vi "Lab Panel V6.00.vi"() -> ()   [LabVIEW 2017] (continued)
                          }
                          frame #1 {
                            n1486 = Bundle(cluster=w2775, "STATUS"="T-RISE PASS") -> (w2777:T4)  [unwired: 2 in]
                            n1487 = local write "RESULT LAB04-1"(TRUE) -> ()
                            n1488 = local write "DISP LAB04-1"(w2777) -> ()
                          }
                        }
                      }
                      frame False {
                      }
                    }
                  }
                }
              }
              frame #7 {
                # "LAB04-2"
                n1489 = Equal?(x=w2780, y=2) -> (x = y?=w2783:bool)
                n1490 = local read "DISP LAB04-2"() -> (w2785:T4)
                n1491 = Unbundle(w2785) -> ("STATUS"=w2786:string)  [unwired: 2 out]
                n1492 = Equal?(x=w2786, y="RUN") -> (x = y?=w2782:bool)
                n1493 = And(x=w2782, y=w2783) -> (x .and. y?=w2781:bool)
                n1494 = case shown="True" w2781 {
                  tunnel: w2785 -> [_ w2789]
                  tunnel: w2779 -> [_ w2792]
                  frame False {
                  }
                  frame True {
                    n1495 = local read "SET LAB04-2"() -> (w2791:T5)
                    n1496 = local read "TDMS LAB04-2"() -> (w2788:refnum<k34>)
                    n1497 = Unbundle(w2789) -> ("CYCLE"=w2793:dbl)  [unwired: 2 out]
                    n1498 = Unbundle(w2791) -> ("T-RISE mins"=w2790:dbl)  [unwired: 4 out]
                    n1499 = Greater Or Equal?(x=w2793, y=w2792) -> (x >= y?=w2794:bool)
                    n1500 = case shown="True" w2794 {
                      tunnel: w2790 -> [w2797 _]
                      tunnel: w2789 -> [w2796 _]
                      tunnel: w2788 -> [w2795 _]
                      frame True {
                        n1501 = stacked-sequence {
                          tunnel: w2797 -> [w2800 _]
                          tunnel: w2796 -> [_ w2805]
                          tunnel: w2795 -> [w2798 _]
                          frame #0 {
                            n1502 = Build Array("T-RISE") -> (w2802:string[])
                            n1503 = Build Array(w2800) -> (w2801:dbl[])
                            n1504 = TDMS Write(0:w2798, 5:"TEST PASS", 7:w2802, 9:w2801) -> (15:w2804:errorcluster)  [unwired: 2 in, 3 out]
                            n1505 = local write "data file error"(w2804) -> ()
                          }
                          frame #1 {
                            n1506 = Bundle(cluster=w2805, "STATUS"="T-RISE PASS") -> (w2807:T4)  [unwired: 2 in]
                            n1507 = local write "RESULT LAB04-2"(TRUE) -> ()
                            n1508 = local write "DISP LAB04-2"(w2807) -> ()
                          }
                        }
                      }
                      frame False {
                      }
                    }
                  }
                }
              }
              frame #8 {
                # "LAB05-1"
                n1509 = Equal?(x=w2810, y=2) -> (x = y?=w2813:bool)
                n1510 = local read "DISP LAB05-1"() -> (w2815:T4)
                n1511 = Unbundle(w2815) -> ("STATUS"=w2816:string)  [unwired: 2 out]
                n1512 = Equal?(x=w2816, y="RUN") -> (x = y?=w2812:bool)
                n1513 = And(x=w2812, y=w2813) -> (x .and. y?=w2811:bool)
                n1514 = case shown="True" w2811 {
                  tunnel: w2815 -> [_ w2819]
                  tunnel: w2809 -> [_ w2822]
                  frame False {
                  }
                  frame True {
                    n1515 = local read "SET LAB05-1"() -> (w2821:T5)
                    n1516 = local read "TDMS LAB05-1"() -> (w2818:refnum<k34>)
                    n1517 = Unbundle(w2819) -> ("CYCLE"=w2823:dbl)  [unwired: 2 out]
                    n1518 = Unbundle(w2821) -> ("T-RISE mins"=w2820:dbl)  [unwired: 4 out]
                    n1519 = Greater Or Equal?(x=w2823, y=w2822) -> (x >= y?=w2824:bool)
                    n1520 = case shown="True" w2824 {
                      tunnel: w2820 -> [w2827 _]
                      tunnel: w2819 -> [w2826 _]
                      tunnel: w2818 -> [w2825 _]
                      frame True {
                        n1521 = stacked-sequence {
                          tunnel: w2827 -> [w2830 _]
                          tunnel: w2826 -> [_ w2835]
                          tunnel: w2825 -> [w2828 _]
                          frame #0 {
                            n1522 = Build Array("T-RISE") -> (w2832:string[])
                            n1523 = Build Array(w2830) -> (w2831:dbl[])
                            n1524 = TDMS Write(0:w2828, 5:"TEST PASS", 7:w2832, 9:w2831) -> (15:w2834:errorcluster)  [unwired: 2 in, 3 out]
                            n1525 = local write "data file error"(w2834) -> ()
                          }
                          frame #1 {
                            n1526 = Bundle(cluster=w2835, "STATUS"="T-RISE PASS") -> (w2837:T4)  [unwired: 2 in]
                            n1527 = local write "RESULT LAB05-1"(TRUE) -> ()
                            n1528 = local write "DISP LAB05-1"(w2837) -> ()
                          }
                        }
                      }
                      frame False {
                      }
                    }
                  }
                }
              }
              frame #9 {
                # "LAB05-2"
                n1529 = Equal?(x=w2840, y=2) -> (x = y?=w2843:bool)
                n1530 = local read "DISP LAB05-2"() -> (w2845:T4)
                n1531 = Unbundle(w2845) -> ("STATUS"=w2846:string)  [unwired: 2 out]
                n1532 = Equal?(x=w2846, y="RUN") -> (x = y?=w2842:bool)
                n1533 = And(x=w2842, y=w2843) -> (x .and. y?=w2841:bool)
                n1534 = case shown="True" w2841 {
                  tunnel: w2845 -> [_ w2849]
                  tunnel: w2839 -> [_ w2852]
                  frame False {
                  }
                  frame True {
                    n1535 = local read "SET LAB05-2"() -> (w2851:T5)
                    n1536 = local read "TDMS LAB05-2"() -> (w2848:refnum<k34>)
                    n1537 = Unbundle(w2849) -> ("CYCLE"=w2853:dbl)  [unwired: 2 out]
                    n1538 = Unbundle(w2851) -> ("T-RISE mins"=w2850:dbl)  [unwired: 4 out]
                    n1539 = Greater Or Equal?(x=w2853, y=w2852) -> (x >= y?=w2854:bool)
                    n1540 = case shown="True" w2854 {
                      tunnel: w2850 -> [w2857 _]
                      tunnel: w2849 -> [w2856 _]
                      tunnel: w2848 -> [w2855 _]
                      frame True {
                        n1541 = stacked-sequence {
                          tunnel: w2857 -> [w2860 _]
                          tunnel: w2856 -> [_ w2865]
                          tunnel: w2855 -> [w2858 _]
                          frame #0 {
                            n1542 = Build Array("T-RISE") -> (w2862:string[])
                            n1543 = Build Array(w2860) -> (w2861:dbl[])
                            n1544 = TDMS Write(0:w2858, 5:"TEST PASS", 7:w2862, 9:w2861) -> (15:w2864:errorcluster)  [unwired: 2 in, 3 out]
                            n1545 = local write "data file error"(w2864) -> ()
                          }
                          frame #1 {
                            n1546 = Bundle(cluster=w2865, "STATUS"="T-RISE PASS") -> (w2867:T4)  [unwired: 2 in]
                            n1547 = local write "RESULT LAB05-2"(TRUE) -> ()
                            n1548 = local write "DISP LAB05-2"(w2867) -> ()
                          }
                        }
                      }
                      frame False {
                      }
                    }
                  }
                }
              }
            }
          }
          frame #7 {
            # "Note : run lab0X-N. RUN LAB0X-N and O/I LAB0X-N   are written to digital I/O in frame 11"
            # "End test & close test files"
            n1549 = local read "MAIL SETTINGS"() -> (w2874:T8)
            n1550 = local read "TO (string):"() -> (w2869:string)
            n1551 = Unbundle(w2874) -> ("OUT SERVER ADDRESS"=w2873:string, "FROM ACCOUNT"=w2872:string)  [unwired: 5 out]
            n1552 = stacked-sequence {
              tunnel: w2884 -> [_ _ _ _ _ _ _ _ _ _]
              tunnel: w2885 -> [_ _ _ _ _ _ _ _ _ _]
              tunnel: w2883 -> [_ _ _ _ _ _ _ _ _ _]
              tunnel: w2882 -> [_ _ _ _ _ _ _ _ _ _]
              tunnel: w2881 -> [_ _ _ _ _ _ _ _ _ _]
              tunnel: w2880 -> [_ _ _ _ _ _ _ _ _ _]
              tunnel: w2879 -> [_ _ _ _ _ _ _ _ _ _]
              tunnel: w2878 -> [_ _ _ _ _ _ _ _ _ _]
              tunnel: w2877 -> [_ _ _ _ _ _ _ _ _ _]
              tunnel: w2876 -> [_ _ _ _ _ _ _ _ _ _]
              tunnel: w2873 -> [w2890 w2942 w2990 w3037 w3084 w3131 w3178 w3225 w3272 w3319]
              tunnel: w2872 -> [w2889 w2941 w2989 w3036 w3083 w3130 w3177 w3224 w3271 w3318]
              tunnel: "Mail Test File To:" -> [w2888 w2940 w2988 w3035 w3082 w3129 w3176 w3223 w3270 w3317]
              tunnel: "Mail Test Fail" -> [w2887 w2939 w2987 w3034 w3081 w3128 w3175 w3222 w3269 w3316]
              frame #0 {
                # "LAB01-1"
                n1553 = local read "DISP LAB01-1"() -> (w2886:T4)
                n1554 = global write "Global display 2.vi" "DISP LAB01-1"(w2886) -> ()
                n1555 = local read "run lab01-1"() -> (w2891:bool)
                n1556 = local read "TDMS LAB01-1"() -> (w2892:refnum<k34>)
                n1557 = Unbundle(w2886) -> ("CYCLE"=w2894:dbl, "STATUS"=w2893:string)  [unwired: 1 out]
                n1558 = case shown="True" w2891 {
                  tunnel: w2894 -> [_ w2900]
                  tunnel: w2886 -> [_ w2902]
                  tunnel: w2893 -> [_ w2899]
                  tunnel: w2892 -> [_ w2901]
                  tunnel: w2890 -> [_ w2898]
                  tunnel: w2889 -> [_ w2897]
                  tunnel: w2888 -> [_ w2896]
                  tunnel: w2887 -> [_ w2895]
                  frame False {
                  }
                  frame True {
                    n1559 = Not Equal?(x=w2899, y="RUN") -> (x != y?=w2903:bool)
                    n1560 = Greater?(x=w2900, y=2.0) -> (0:w2905:bool)
                    n1561 = And(x=w2905, y=w2903) -> (x .and. y?=w2904:bool)
                    n1562 = case shown="True" w2904 {
                      tunnel: w2902 -> [_ w2915]
                      tunnel: w2901 -> [_ w2914]
                      tunnel: w2900 -> [_ w2913]
                      tunnel: w2899 -> [_ w2912]
                      tunnel: w2898 -> [_ w2911]
                      tunnel: w2897 -> [_ w2910]
                      tunnel: w2896 -> [_ w2909]
                      tunnel: w2895 -> [_ w2908]
                      frame False {
                      }
                      frame True {
                        n1563 = stacked-sequence {
                          tunnel: w2915 -> [w2919 _ _]
                          tunnel: w2914 -> [_ w2921 _]
                          tunnel: w2913 -> [_ _ _]
                          tunnel: w2912 -> [_ _ w2927]
                          tunnel: w2911 -> [_ _ w2926]
                          tunnel: w2910 -> [_ _ w2925]
                          tunnel: w2909 -> [_ _ w2924]
                          tunnel: w2908 -> [_ _ w2923]
                          frame #0 {
                            w2916 = FALSE
                            n1564 = local write "mail control"("END") -> ()
                            n1565 = Bundle(cluster=w2919) -> (w2918:T4)  [unwired: 3 in]
                            n1566 = local write "DISP LAB01-1"(w2918) -> ()
                            n1567 = local write "O/I  LAB01-1"(w2916) -> ()
                            n1568 = local write "run lab01-1"(w2916) -> ()
                            n1569 = local write "RUN LAB01-1"(w2916) -> ()
                          }
                          frame #1 {
                            n1570 = TDMS Close(11:w2921) -> (0:w2920:errorcluster)  [unwired: 1 in, 1 out]
                            n1571 = local write "data file error"(w2920) -> ()
                          }
                          frame #2 {
                            n1572 = stacked-sequence {
                              tunnel: "LAB01-1" -> [w2929 w2932 _]
                              tunnel: w2927 -> [_ w2938 _]
                              tunnel: w2926 -> [_ w2937 _]
                              tunnel: w2925 -> [_ w2936 _]
                              tunnel: w2924 -> [_ w2935 _]
                              tunnel: w2923 -> [_ w2934 _]
                              frame #0 {
                                n1573 = call "sub vi - defrag tdms v1.vi"("panel id"=w2929) -> ("error out"=w2928:errorcluster)  [unwired: 10 in]
                                n1574 = local write "data file error"(w2928) -> ()
                              }
                              frame #1 {
                                n1575 = Bundle By Name(cluster=T23 {"status"="", "mail server"="", "mail from"="", "mail to"="", "mail file"=FALSE} ("Input Cluster"), "status"=w2938, "mail server"=w2937, "mail from"=w2936, "mail to"=w2935, "mail file"=w2934) -> (w2931:T23)
                                n1576 = call "Save data file (pass-fail) v5.vi"("Input Cluster"=w2931, "panel id"=w2932) -> ("network file save error"=w2933:errorcluster)  [unwired: 8 in, 1 out]
                                n1577 = local write "data file error"(w2933) -> ()
                              }
                              frame #2 {
                              }
                            }
                          }
                        }
                      }
                    }
                  }
                }
              }
              frame #1 {
                # "LAB01-2"
                n1578 = local read "run lab01-2"() -> (w2943:bool)
                n1579 = case shown="True" w2943 {
                  tunnel: w2942 -> [_ w2948]
                  tunnel: w2941 -> [_ w2947]
                  tunnel: w2940 -> [_ w2946]
                  tunnel: w2939 -> [_ w2945]
                  frame False {
                  }
                  frame True {
                    n1580 = local read "DISP LAB01-2"() -> (w2944:T4)
                    n1581 = global write "Global display 2.vi" "DISP LAB01-2"(w2944) -> ()
                    n1582 = local read "TDMS LAB01-2"() -> (w2955:refnum<k34>)
                    n1583 = Unbundle(w2944) -> ("CYCLE"=w2950:dbl, "STATUS"=w2949:string)  [unwired: 1 out]
                    n1584 = Not Equal?(x=w2949, y="RUN") -> (x != y?=w2952:bool)
                    n1585 = Greater?(x=w2950, y=2.0) -> (0:w2953:bool)
                    n1586 = And(x=w2953, y=w2952) -> (x .and. y?=w2951:bool)
                    n1587 = case shown="True" w2951 {
                      tunnel: w2944 -> [_ w2964]
                      tunnel: w2955 -> [_ w2963]
                      tunnel: w2950 -> [_ w2962]
                      tunnel: w2949 -> [_ w2961]
                      tunnel: w2948 -> [_ w2960]
                      tunnel: w2947 -> [_ w2959]
                      tunnel: w2946 -> [_ w2958]
                      tunnel: w2945 -> [_ w2957]
                      frame False {
                      }
                      frame True {
                        n1588 = stacked-sequence {
                          tunnel: w2964 -> [w2967 _ _]
                          tunnel: w2963 -> [_ w2969 _]
                          tunnel: w2962 -> [_ _ _]
                          tunnel: w2961 -> [_ _ w2975]
                          tunnel: w2960 -> [_ _ w2974]
                          tunnel: w2959 -> [_ _ w2973]
                          tunnel: w2958 -> [_ _ w2972]
                          tunnel: w2957 -> [_ _ w2971]
                          frame #0 {
                            w2965 = FALSE
                            n1589 = local write "mail control"("END") -> ()
                            n1590 = Bundle(cluster=w2967) -> (w2968:T4)  [unwired: 3 in]
                            n1591 = local write "RUN LAB01-2"(w2965) -> ()
                            n1592 = local write "run lab01-2"(w2965) -> ()
                            n1593 = local write "O/I  LAB01-2"(w2965) -> ()
                            n1594 = local write "DISP LAB01-2"(w2968) -> ()
                          }
                          frame #1 {
                            n1595 = TDMS Close(11:w2969) -> (0:w2970:errorcluster)  [unwired: 1 in, 1 out]
                            n1596 = local write "data file error"(w2970) -> ()
                          }
                          frame #2 {
                            n1597 = stacked-sequence {
                              tunnel: "LAB01-2" -> [w2978 w2979]
                              tunnel: w2975 -> [_ w2984]
                              tunnel: w2974 -> [_ w2983]
                              tunnel: w2973 -> [_ w2982]
                              tunnel: w2972 -> [_ w2981]
                              tunnel: w2971 -> [_ w2980]
                              frame #0 {
                                n1598 = call "sub vi - defrag tdms v1.vi"("panel id"=w2978) -> ("error out"=w2977:errorcluster)  [unwired: 10 in]
                                n1599 = local write "data file error"(w2977) -> ()
                              }
                              frame #1 {
                                n1600 = Bundle("STATUS"=w2984, "OUT SERVER ADDRESS"=w2983, "FROM ACCOUNT"=w2982, "Mail Test File To:"=w2981, "Mail Test Fail"=w2980) -> (w2986:T29)  [unwired: 1 in]
                                n1601 = call "Save data file (pass-fail) v5.vi"("Input Cluster"=w2986, "panel id"=w2979) -> ("network file save error"=w2985:errorcluster)  [unwired: 8 in, 1 out]
                                n1602 = local write "data file error"(w2985) -> ()
                              }
                            }
                          }
                        }
                      }
                    }
                  }
                }
              }
              frame #2 {
                # "LAB02-1"
                n1603 = local read "run lab02-1"() -> (w2991:bool)
                n1604 = case shown="True" w2991 {
                  tunnel: w2990 -> [_ w2996]
                  tunnel: w2989 -> [_ w2995]
                  tunnel: w2988 -> [_ w2994]
                  tunnel: w2987 -> [_ w2993]
                  frame False {
                  }
                  frame True {
                    n1605 = local read "DISP LAB02-1"() -> (w2992:T4)
                    n1606 = global write "Global display 2.vi" "DISP LAB02-1"(w2992) -> ()
                    n1607 = Unbundle(w2992) -> ("CYCLE"=w3000:dbl, "STATUS"=w2997:string)  [unwired: 1 out]
                    n1608 = local read "TDMS LAB02-1"() -> (w3003:refnum<k34>)
                    n1609 = Not Equal?(x=w2997, y="RUN") -> (x != y?=w2999:bool)
                    n1610 = Greater?(x=w3000, y=2.0) -> (0:w3001:bool)
                    n1611 = And(x=w3001, y=w2999) -> (x .and. y?=w2998:bool)
                    n1612 = case shown="True" w2998 {
                      tunnel: w2992 -> [_ w3011]
                      tunnel: w3003 -> [_ w3010]
                      tunnel: w2997 -> [_ w3009]
                      tunnel: w2996 -> [_ w3008]
                      tunnel: w2995 -> [_ w3007]
                      tunnel: w2994 -> [_ w3006]
                      tunnel: w2993 -> [_ w3005]
                      frame False {
                      }
                      frame True {
                        n1613 = stacked-sequence {
                          tunnel: w3011 -> [w3014 _ _]
                          tunnel: w3010 -> [_ w3016 _]
                          tunnel: w3009 -> [_ _ w3022]
                          tunnel: w3008 -> [_ _ w3021]
                          tunnel: w3007 -> [_ _ w3020]
                          tunnel: w3006 -> [_ _ w3019]
                          tunnel: w3005 -> [_ _ w3018]
                          frame #0 {
                            w3012 = FALSE
                            n1614 = local write "mail control"("END") -> ()
                            n1615 = Bundle(cluster=w3014) -> (w3015:T4)  [unwired: 3 in]
                            n1616 = local write "O/I  LAB02-1"(w3012) -> ()
                            n1617 = local write "RUN LAB02-1"(w3012) -> ()
                            n1618 = local write "run lab02-1"(w3012) -> ()
                            n1619 = local write "DISP LAB02-1"(w3015) -> ()
                          }
                          frame #1 {
                            n1620 = TDMS Close(11:w3016) -> (0:w3017:errorcluster)  [unwired: 1 in, 1 out]
                            n1621 = local write "data file error"(w3017) -> ()
                          }
                          frame #2 {
                            n1622 = stacked-sequence {
                              tunnel: "LAB02-1" -> [w3025 w3032]
                              tunnel: w3022 -> [_ w3030]
                              tunnel: w3021 -> [_ w3029]
                              tunnel: w3020 -> [_ w3028]
                              tunnel: w3019 -> [_ w3027]
                              tunnel: w3018 -> [_ w3026]
                              frame #0 {
                                n1623 = call "sub vi - defrag tdms v1.vi"("panel id"=w3025) -> ("error out"=w3024:errorcluster)  [unwired: 10 in]
                                n1624 = local write "data file error"(w3024) -> ()
                              }
                              frame #1 {
                                n1625 = Bundle("STATUS"=w3030, "OUT SERVER ADDRESS"=w3029, "FROM ACCOUNT"=w3028, "Mail Test File To:"=w3027, "Mail Test Fail"=w3026) -> (w3031:T29)  [unwired: 1 in]
                                n1626 = call "Save data file (pass-fail) v5.vi"("Input Cluster"=w3031, "panel id"=w3032) -> ("network file save error"=w3033:errorcluster)  [unwired: 8 in, 1 out]
                                n1627 = local write "data file error"(w3033) -> ()
                              }
                            }
                          }
                        }
                      }
                    }
                  }
                }
              }
              frame #3 {
                # "LAB02-2"
                n1628 = local read "run lab02-2"() -> (w3038:bool)
                n1629 = case shown="True" w3038 {
                  tunnel: w3037 -> [_ w3044]
                  tunnel: w3036 -> [_ w3043]
                  tunnel: w3035 -> [_ w3042]
                  tunnel: w3034 -> [_ w3041]
                  frame False {
                  }
                  frame True {
                    n1630 = local read "DISP LAB02-2"() -> (w3040:T4)
                    n1631 = global write "Global display 2.vi" "DISP LAB02-2"(w3040) -> ()
                    n1632 = local read "TDMS LAB02-2"() -> (w3050:refnum<k34>)
                    n1633 = Unbundle(w3040) -> ("CYCLE"=w3039:dbl, "STATUS"=w3045:string)  [unwired: 1 out]
                    n1634 = Not Equal?(x=w3045, y="RUN") -> (x != y?=w3047:bool)
                    n1635 = Greater?(x=w3039, y=2.0) -> (0:w3048:bool)
                    n1636 = And(x=w3048, y=w3047) -> (x .and. y?=w3046:bool)
                    n1637 = case shown="True" w3046 {
                      tunnel: w3040 -> [_ w3058]
                      tunnel: w3050 -> [_ w3057]
                      tunnel: w3045 -> [_ w3056]
                      tunnel: w3044 -> [_ w3055]
                      tunnel: w3043 -> [_ w3054]
                      tunnel: w3042 -> [_ w3053]
                      tunnel: w3041 -> [_ w3052]
                      frame False {
                      }
                      frame True {
                        n1638 = stacked-sequence {
                          tunnel: w3058 -> [w3061 _ _]
                          tunnel: w3057 -> [_ w3063 _]
                          tunnel: w3056 -> [_ _ w3069]
                          tunnel: w3055 -> [_ _ w3068]
                          tunnel: w3054 -> [_ _ w3067]
                          tunnel: w3053 -> [_ _ w3066]
                          tunnel: w3052 -> [_ _ w3065]
                          frame #0 {
                            w3059 = FALSE
                            n1639 = local write "mail control"("END") -> ()
                            n1640 = Bundle(cluster=w3061) -> (w3062:T4)  [unwired: 3 in]
                            n1641 = local write "O/I  LAB02-2"(w3059) -> ()
                            n1642 = local write "run lab02-2"(w3059) -> ()
                            n1643 = local write "RUN LAB02-2"(w3059) -> ()
                            n1644 = local write "DISP LAB02-2"(w3062) -> ()
                          }
                          frame #1 {
                            n1645 = TDMS Close(11:w3063) -> (0:w3064:errorcluster)  [unwired: 1 in, 1 out]
                            n1646 = local write "data file error"(w3064) -> ()
                          }
                          frame #2 {
                            n1647 = stacked-sequence {
                              tunnel: "LAB02-2" -> [w3072 w3078]
                              tunnel: w3069 -> [_ w3077]
                              tunnel: w3068 -> [_ w3076]
                              tunnel: w3067 -> [_ w3075]
                              tunnel: w3066 -> [_ w3074]
                              tunnel: w3065 -> [_ w3073]
                              frame #0 {
                                n1648 = call "sub vi - defrag tdms v1.vi"("panel id"=w3072) -> ("error out"=w3071:errorcluster)  [unwired: 10 in]
                                n1649 = local write "data file error"(w3071) -> ()
                              }
                              frame #1 {
                                n1650 = Bundle("STATUS"=w3077, "OUT SERVER ADDRESS"=w3076, "FROM ACCOUNT"=w3075, "Mail Test File To:"=w3074, "Mail Test Fail"=w3073) -> (w3080:T29)  [unwired: 1 in]
                                n1651 = call "Save data file (pass-fail) v5.vi"("Input Cluster"=w3080, "panel id"=w3078) -> ("network file save error"=w3079:errorcluster)  [unwired: 8 in, 1 out]
                                n1652 = local write "data file error"(w3079) -> ()
                              }
                            }
                          }
                        }
                      }
                    }
                  }
                }
              }
              frame #4 {
                # "LAB03-1"
                n1653 = local read "run lab03-1"() -> (w3085:bool)
                n1654 = case shown="True" w3085 {
                  tunnel: w3084 -> [_ w3090]
                  tunnel: w3083 -> [_ w3089]
                  tunnel: w3082 -> [_ w3088]
                  tunnel: w3081 -> [_ w3087]
                  frame False {
                  }
                  frame True {
                    n1655 = local read "DISP LAB03-1"() -> (w3086:T4)
                    n1656 = local read "TDMS LAB03-1"() -> (w3097:refnum<k34>)
                    n1657 = global write "Global display 2.vi" "DISP LAB03-1"(w3086) -> ()
                    n1658 = Unbundle(w3086) -> ("CYCLE"=w3094:dbl, "STATUS"=w3091:string)  [unwired: 1 out]
                    n1659 = Not Equal?(x=w3091, y="RUN") -> (x != y?=w3093:bool)
                    n1660 = Greater?(x=w3094, y=2.0) -> (0:w3095:bool)
                    n1661 = And(x=w3095, y=w3093) -> (x .and. y?=w3092:bool)
                    n1662 = case shown="True" w3092 {
                      tunnel: w3086 -> [_ w3105]
                      tunnel: w3097 -> [_ w3104]
                      tunnel: w3091 -> [_ w3103]
                      tunnel: w3090 -> [_ w3102]
                      tunnel: w3089 -> [_ w3101]
                      tunnel: w3088 -> [_ w3100]
                      tunnel: w3087 -> [_ w3099]
                      frame False {
                      }
                      frame True {
                        n1663 = stacked-sequence {
                          tunnel: w3105 -> [w3108 _ _]
                          tunnel: w3104 -> [_ w3110 _]
                          tunnel: w3103 -> [_ _ w3116]
                          tunnel: w3102 -> [_ _ w3115]
                          tunnel: w3101 -> [_ _ w3114]
                          tunnel: w3100 -> [_ _ w3113]
                          tunnel: w3099 -> [_ _ w3112]
                          frame #0 {
                            w3106 = FALSE
                            n1664 = local write "mail control"("END") -> ()
                            n1665 = Bundle(cluster=w3108) -> (w3109:T4)  [unwired: 3 in]
                            n1666 = local write "O/I  LAB03-1"(w3106) -> ()
                            n1667 = local write "run lab03-1"(w3106) -> ()
                            n1668 = local write "RUN LAB03-1"(w3106) -> ()
                            n1669 = local write "DISP LAB03-1"(w3109) -> ()
                          }
                          frame #1 {
                            n1670 = TDMS Close(11:w3110) -> (0:w3111:errorcluster)  [unwired: 1 in, 1 out]
                            n1671 = local write "data file error"(w3111) -> ()
                          }
                          frame #2 {
                            n1672 = stacked-sequence {
                              tunnel: "LAB03-1" -> [w3119 w3125]
                              tunnel: w3116 -> [_ w3124]
                              tunnel: w3115 -> [_ w3123]
                              tunnel: w3114 -> [_ w3122]
                              tunnel: w3113 -> [_ w3121]
                              tunnel: w3112 -> [_ w3120]
                              frame #0 {
                                n1673 = call "sub vi - defrag tdms v1.vi"("panel id"=w3119) -> ("error out"=w3118:errorcluster)  [unwired: 10 in]
                                n1674 = local write "data file error"(w3118) -> ()
                              }
                              frame #1 {
                                n1675 = Bundle("STATUS"=w3124, "OUT SERVER ADDRESS"=w3123, "FROM ACCOUNT"=w3122, "Mail Test File To:"=w3121, "Mail Test Fail"=w3120) -> (w3127:T29)  [unwired: 1 in]
                                n1676 = call "Save data file (pass-fail) v5.vi"("Input Cluster"=w3127, "panel id"=w3125) -> ("network file save error"=w3126:errorcluster)  [unwired: 8 in, 1 out]
                                n1677 = local write "data file error"(w3126) -> ()
                              }
                            }
                          }
                        }
                      }
                    }
                  }
                }
              }
              frame #5 {
                # "LAB03-2"
                n1678 = local read "run lab03-2"() -> (w3132:bool)
                n1679 = case shown="True" w3132 {
                  tunnel: w3131 -> [_ w3137]
                  tunnel: w3130 -> [_ w3136]
                  tunnel: w3129 -> [_ w3135]
                  tunnel: w3128 -> [_ w3134]
                  frame False {
                  }
                  frame True {
                    n1680 = local read "DISP LAB03-2"() -> (w3133:T4)
                    n1681 = global write "Global display 2.vi" "DISP LAB03-2"(w3133) -> ()
                    n1682 = Unbundle(w3133) -> ("CYCLE"=w3141:dbl, "STATUS"=w3138:string)  [unwired: 1 out]
                    n1683 = local read "TDMS LAB03-2"() -> (w3144:refnum<k34>)
                    n1684 = Not Equal?(x=w3138, y="RUN") -> (x != y?=w3140:bool)
                    n1685 = Greater?(x=w3141, y=2.0) -> (0:w3142:bool)
                    n1686 = And(x=w3142, y=w3140) -> (x .and. y?=w3139:bool)
                    n1687 = case shown="True" w3139 {
                      tunnel: w3133 -> [_ w3152]
                      tunnel: w3144 -> [_ w3151]
                      tunnel: w3138 -> [_ w3150]
                      tunnel: w3137 -> [_ w3149]
                      tunnel: w3136 -> [_ w3148]
                      tunnel: w3135 -> [_ w3147]
                      tunnel: w3134 -> [_ w3146]
                      frame False {
                      }
                      frame True {
                        n1688 = stacked-sequence {
                          tunnel: w3152 -> [w3155 _ _]
                          tunnel: w3151 -> [_ w3157 _]
                          tunnel: w3150 -> [_ _ w3163]
                          tunnel: w3149 -> [_ _ w3162]
                          tunnel: w3148 -> [_ _ w3161]
                          tunnel: w3147 -> [_ _ w3160]
                          tunnel: w3146 -> [_ _ w3159]
                          frame #0 {
                            w3153 = FALSE
                            n1689 = local write "mail control"("END") -> ()
                            n1690 = Bundle(cluster=w3155) -> (w3156:T4)  [unwired: 3 in]
                            n1691 = local write "RUN LAB03-2"(w3153) -> ()
                            n1692 = local write "O/I  LAB03-2"(w3153) -> ()
                            n1693 = local write "DISP LAB03-2"(w3156) -> ()
                            n1694 = local write "run lab03-2"(w3153) -> ()
                          }
                          frame #1 {
                            n1695 = TDMS Close(11:w3157) -> (0:w3158:errorcluster)  [unwired: 1 in, 1 out]
                            n1696 = local write "data file error"(w3158) -> ()
                          }
                          frame #2 {
                            n1697 = stacked-sequence {
                              tunnel: "LAB03-2" -> [w3166 w3167]
                              tunnel: w3163 -> [_ w3172]
                              tunnel: w3162 -> [_ w3171]
                              tunnel: w3161 -> [_ w3170]
                              tunnel: w3160 -> [_ w3169]
                              tunnel: w3159 -> [_ w3168]
                              frame #0 {
                                n1698 = call "sub vi - defrag tdms v1.vi"("panel id"=w3166) -> ("error out"=w3165:errorcluster)  [unwired: 10 in]
                                n1699 = local write "data file error"(w3165) -> ()
                              }
                              frame #1 {
                                n1700 = Bundle("STATUS"=w3172, "OUT SERVER ADDRESS"=w3171, "FROM ACCOUNT"=w3170, "Mail Test File To:"=w3169, "Mail Test Fail"=w3168) -> (w3174:T29)  [unwired: 1 in]
                                n1701 = call "Save data file (pass-fail) v5.vi"("Input Cluster"=w3174, "panel id"=w3167) -> ("network file save error"=w3173:errorcluster)  [unwired: 8 in, 1 out]
                                n1702 = local write "data file error"(w3173) -> ()
                              }
                            }
                          }
                        }
                      }
                    }
                  }
                }
              }
              frame #6 {
                # "LAB04-1"
                n1703 = local read "run lab04-1"() -> (w3179:bool)
                n1704 = case shown="True" w3179 {
                  tunnel: w3178 -> [_ w3184]
                  tunnel: w3177 -> [_ w3183]
                  tunnel: w3176 -> [_ w3182]
                  tunnel: w3175 -> [_ w3181]
                  frame False {
                  }
                  frame True {
                    n1705 = local read "DISP LAB04-1"() -> (w3180:T4)
                    n1706 = Unbundle(w3180) -> ("CYCLE"=w3188:dbl, "STATUS"=w3185:string)  [unwired: 1 out]
                    n1707 = local read "TDMS LAB04-1"() -> (w3191:refnum<k34>)
                    n1708 = global write "Global display 2.vi" "DISP LAB04-1"(w3180) -> ()
                    n1709 = Not Equal?(x=w3185, y="RUN") -> (x != y?=w3187:bool)
                    n1710 = Greater?(x=w3188, y=2.0) -> (0:w3189:bool)
                    n1711 = And(x=w3189, y=w3187) -> (x .and. y?=w3186:bool)
                    n1712 = case shown="True" w3186 {
                      tunnel: w3180 -> [_ w3199]
                      tunnel: w3191 -> [_ w3198]
                      tunnel: w3185 -> [_ w3197]
                      tunnel: w3184 -> [_ w3196]
                      tunnel: w3183 -> [_ w3195]
                      tunnel: w3182 -> [_ w3194]
                      tunnel: w3181 -> [_ w3193]
                      frame False {
                      }
                      frame True {
                        n1713 = stacked-sequence {
                          tunnel: w3199 -> [w3202 _ _]
                          tunnel: w3198 -> [_ w3204 _]
                          tunnel: w3197 -> [_ _ w3210]
                          tunnel: w3196 -> [_ _ w3209]
                          tunnel: w3195 -> [_ _ w3208]
                          tunnel: w3194 -> [_ _ w3207]
                          tunnel: w3193 -> [_ _ w3206]
                          frame #0 {
                            w3200 = FALSE
                            n1714 = local write "mail control"("END") -> ()
                            n1715 = Bundle(cluster=w3202) -> (w3203:T4)  [unwired: 3 in]
                            n1716 = local write "RUN LAB04-1"(w3200) -> ()
                            n1717 = local write "O/I  LAB04-1"(w3200) -> ()
                            n1718 = local write "run lab04-1"(w3200) -> ()
                            n1719 = local write "DISP LAB04-1"(w3203) -> ()
                          }
                          frame #1 {
                            n1720 = TDMS Close(11:w3204) -> (0:w3205:errorcluster)  [unwired: 1 in, 1 out]
                            n1721 = local write "data file error"(w3205) -> ()
                          }
                          frame #2 {
                            n1722 = stacked-sequence {
                              tunnel: "LAB04-1" -> [w3213 w3214]
                              tunnel: w3210 -> [_ w3219]
                              tunnel: w3209 -> [_ w3218]
                              tunnel: w3208 -> [_ w3217]
                              tunnel: w3207 -> [_ w3216]
                              tunnel: w3206 -> [_ w3215]
                              frame #0 {
                                n1723 = call "sub vi - defrag tdms v1.vi"("panel id"=w3213) -> ("error out"=w3212:errorcluster)  [unwired: 10 in]
                                n1724 = local write "data file error"(w3212) -> ()
                              }
                              frame #1 {
                                n1725 = Bundle("STATUS"=w3219, "OUT SERVER ADDRESS"=w3218, "FROM ACCOUNT"=w3217, "Mail Test File To:"=w3216, "Mail Test Fail"=w3215) -> (w3221:T29)  [unwired: 1 in]
                                n1726 = call "Save data file (pass-fail) v5.vi"("Input Cluster"=w3221, "panel id"=w3214) -> ("network file save error"=w3220:errorcluster)  [unwired: 8 in, 1 out]
                                n1727 = local write "data file error"(w3220) -> ()
                              }
                            }
                          }
                        }
                      }
                    }
                  }
                }
              }
              frame #7 {
                # "LAB04-2"
                n1728 = local read "run lab04-2"() -> (w3226:bool)
                n1729 = case shown="True" w3226 {
                  tunnel: w3225 -> [_ w3231]
                  tunnel: w3224 -> [_ w3230]
                  tunnel: w3223 -> [_ w3229]
                  tunnel: w3222 -> [_ w3228]
                  frame False {
                  }
                  frame True {
                    n1730 = local read "DISP LAB04-2"() -> (w3227:T4)
                    n1731 = Unbundle(w3227) -> ("CYCLE"=w3235:dbl, "STATUS"=w3232:string)  [unwired: 1 out]
                    n1732 = global write "Global display 2.vi" "DISP LAB04-2"(w3227) -> ()
                    n1733 = Not Equal?(x=w3232, y="RUN") -> (x != y?=w3234:bool)
                    n1734 = local read "TDMS LAB04-2"() -> (w3238:refnum<k34>)
                    n1735 = Greater?(x=w3235, y=2.0) -> (0:w3236:bool)
                    n1736 = And(x=w3236, y=w3234) -> (x .and. y?=w3233:bool)
                    n1737 = case shown="True" w3233 {
                      tunnel: w3227 -> [_ w3246]
                      tunnel: w3238 -> [_ w3245]
                      tunnel: w3232 -> [_ w3244]
                      tunnel: w3231 -> [_ w3243]
                      tunnel: w3230 -> [_ w3242]
                      tunnel: w3229 -> [_ w3241]
                      tunnel: w3228 -> [_ w3240]
                      frame False {
                      }
                      frame True {
                        n1738 = stacked-sequence {
                          tunnel: w3246 -> [w3249 _ _]
                          tunnel: w3245 -> [_ w3251 _]
                          tunnel: w3244 -> [_ _ w3257]
                          tunnel: w3243 -> [_ _ w3256]
                          tunnel: w3242 -> [_ _ w3255]
                          tunnel: w3241 -> [_ _ w3254]
                          tunnel: w3240 -> [_ _ w3253]
                          frame #0 {
                            w3247 = FALSE
                            n1739 = local write "mail control"("END") -> ()
                            n1740 = Bundle(cluster=w3249) -> (w3250:T4)  [unwired: 3 in]
                            n1741 = local write "O/I  LAB04-2"(w3247) -> ()
                            n1742 = local write "RUN LAB04-2"(w3247) -> ()
                            n1743 = local write "run lab04-2"(w3247) -> ()
                            n1744 = local write "DISP LAB04-2"(w3250) -> ()
                          }
                          frame #1 {
                            n1745 = TDMS Close(11:w3251) -> (0:w3252:errorcluster)  [unwired: 1 in, 1 out]
                            n1746 = local write "data file error"(w3252) -> ()
                          }
                          frame #2 {
                            n1747 = stacked-sequence {
                              tunnel: "LAB04-2" -> [w3260 w3261]
                              tunnel: w3257 -> [_ w3266]
                              tunnel: w3256 -> [_ w3265]
                              tunnel: w3255 -> [_ w3264]
                              tunnel: w3254 -> [_ w3263]
                              tunnel: w3253 -> [_ w3262]
                              frame #0 {
                                n1748 = call "sub vi - defrag tdms v1.vi"("panel id"=w3260) -> ("error out"=w3259:errorcluster)  [unwired: 10 in]
                                n1749 = local write "data file error"(w3259) -> ()
                              }
                              frame #1 {
                                n1750 = Bundle("STATUS"=w3266, "OUT SERVER ADDRESS"=w3265, "FROM ACCOUNT"=w3264, "Mail Test File To:"=w3263, "Mail Test Fail"=w3262) -> (w3268:T29)  [unwired: 1 in]
                                n1751 = call "Save data file (pass-fail) v5.vi"("Input Cluster"=w3268, "panel id"=w3261) -> ("network file save error"=w3267:errorcluster)  [unwired: 8 in, 1 out]
                                n1752 = local write "data file error"(w3267) -> ()
                              }
                            }
                          }
                        }
                      }
                    }
                  }
                }
              }
              frame #8 {
                # "LAB05-1"
                n1753 = local read "run lab05-1"() -> (w3273:bool)
                n1754 = case shown="True" w3273 {
                  tunnel: w3272 -> [_ w3278]
                  tunnel: w3271 -> [_ w3277]
                  tunnel: w3270 -> [_ w3276]
                  tunnel: w3269 -> [_ w3275]
                  frame False {
                  }
                  frame True {
                    n1755 = local read "DISP LAB05-1"() -> (w3274:T4)
                    n1756 = Unbundle(w3274) -> ("CYCLE"=w3282:dbl, "STATUS"=w3279:string)  [unwired: 1 out]
                    n1757 = global write "Global display 2.vi" "DISP LAB05-1"(w3274) -> ()
                    n1758 = Not Equal?(x=w3279, y="RUN") -> (x != y?=w3281:bool)
                    n1759 = local read "TDMS LAB05-1"() -> (w3285:refnum<k34>)
                    n1760 = Greater?(x=w3282, y=2.0) -> (0:w3283:bool)
                    n1761 = And(x=w3283, y=w3281) -> (x .and. y?=w3280:bool)
                    n1762 = case shown="True" w3280 {
                      tunnel: w3274 -> [_ w3293]
                      tunnel: w3285 -> [_ w3292]
                      tunnel: w3279 -> [_ w3291]
                      tunnel: w3278 -> [_ w3290]
                      tunnel: w3277 -> [_ w3289]
                      tunnel: w3276 -> [_ w3288]
                      tunnel: w3275 -> [_ w3287]
                      frame False {
                      }
                      frame True {
                        n1763 = stacked-sequence {
                          tunnel: w3293 -> [w3296 _ _]
                          tunnel: w3292 -> [_ w3298 _]
                          tunnel: w3291 -> [_ _ w3304]
                          tunnel: w3290 -> [_ _ w3303]
                          tunnel: w3289 -> [_ _ w3302]
                          tunnel: w3288 -> [_ _ w3301]
                          tunnel: w3287 -> [_ _ w3300]
                          frame #0 {
                            w3294 = FALSE
                            n1764 = local write "mail control"("END") -> ()
                            n1765 = Bundle(cluster=w3296) -> (w3297:T4)  [unwired: 3 in]
                            n1766 = local write "O/I  LAB05-1"(w3294) -> ()
                            n1767 = local write "RUN LAB05-1"(w3294) -> ()
                            n1768 = local write "run lab05-1"(w3294) -> ()
                            n1769 = local write "DISP LAB05-1"(w3297) -> ()
                          }
                          frame #1 {
                            n1770 = TDMS Close(11:w3298) -> (0:w3299:errorcluster)  [unwired: 1 in, 1 out]
                            n1771 = local write "data file error"(w3299) -> ()
                          }
                          frame #2 {
                            n1772 = stacked-sequence {
                              tunnel: "LAB05-1" -> [w3307 w3313]
                              tunnel: w3304 -> [_ w3312]
                              tunnel: w3303 -> [_ w3311]
                              tunnel: w3302 -> [_ w3310]
                              tunnel: w3301 -> [_ w3309]
                              tunnel: w3300 -> [_ w3308]
                              frame #0 {
                                n1773 = call "sub vi - defrag tdms v1.vi"("panel id"=w3307) -> ("error out"=w3306:errorcluster)  [unwired: 10 in]
                                n1774 = local write "data file error"(w3306) -> ()
                              }
                              frame #1 {
                                n1775 = Bundle("STATUS"=w3312, "OUT SERVER ADDRESS"=w3311, "FROM ACCOUNT"=w3310, "Mail Test File To:"=w3309, "Mail Test Fail"=w3308) -> (w3315:T29)  [unwired: 1 in]
                                n1776 = call "Save data file (pass-fail) v5.vi"("Input Cluster"=w3315, "panel id"=w3313) -> ("network file save error"=w3314:errorcluster)  [unwired: 8 in, 1 out]
                                n1777 = local write "data file error"(w3314) -> ()
                              }
                            }
                          }
                        }
                      }
                    }
                  }
                }
              }
              frame #9 {
                # "LAB05-2"
                n1778 = local read "run lab05-2"() -> (w3320:bool)
                n1779 = case shown="True" w3320 {
                  tunnel: w3319 -> [_ w3325]
                  tunnel: w3318 -> [_ w3324]
                  tunnel: w3317 -> [_ w3323]
                  tunnel: w3316 -> [_ w3322]
                  frame False {
                  }
                  frame True {
                    n1780 = local read "DISP LAB05-2"() -> (w3321:T4)
                    n1781 = Unbundle(w3321) -> ("CYCLE"=w3329:dbl, "STATUS"=w3326:string)  [unwired: 1 out]
                    n1782 = global write "Global display 2.vi" "DISP LAB05-2"(w3321) -> ()
                    n1783 = Not Equal?(x=w3326, y="RUN") -> (x != y?=w3328:bool)
                    n1784 = local read "TDMS LAB05-2"() -> (w3332:refnum<k34>)
                    n1785 = Greater?(x=w3329, y=2.0) -> (0:w3330:bool)
                    n1786 = And(x=w3330, y=w3328) -> (x .and. y?=w3327:bool)
                    n1787 = case shown="True" w3327 {
                      tunnel: w3321 -> [_ w3340]
                      tunnel: w3332 -> [_ w3339]
                      tunnel: w3326 -> [_ w3338]
                      tunnel: w3325 -> [_ w3337]
                      tunnel: w3324 -> [_ w3336]
                      tunnel: w3323 -> [_ w3335]
                      tunnel: w3322 -> [_ w3334]
                      frame False {
                      }
                      frame True {
                        n1788 = stacked-sequence {
                          tunnel: w3340 -> [w3343 _ _]
                          tunnel: w3339 -> [_ w3345 _]
                          tunnel: w3338 -> [_ _ w3351]
                          tunnel: w3337 -> [_ _ w3350]
                          tunnel: w3336 -> [_ _ w3349]
                          tunnel: w3335 -> [_ _ w3348]
                          tunnel: w3334 -> [_ _ w3347]
                          frame #0 {
                            w3341 = FALSE
